vi "24HP_Convert serial string to Eng vals.vi"(0 "Serial buffer string (excluding FrameChar)":string) -> (2 "Pressures":sgl[][](graph), 3 "T_external (°C)":sgl format="%#_4f", 4 "T_board (°C)":sgl format="%#_4f", 6 "P_atmos (mbar)":sgl format="%#_4f", 8 "RH (%)":sgl format="%#_4f", 10 "a_xyz (g)":sgl[](array[numeric]), 13 "All vals":sgl[](array[numeric]), 14 "Status bytes":u8[](array[numeric]), 15 "w_xyz (deg/s)":sgl[](array[numeric]))   [LabVIEW 2020]
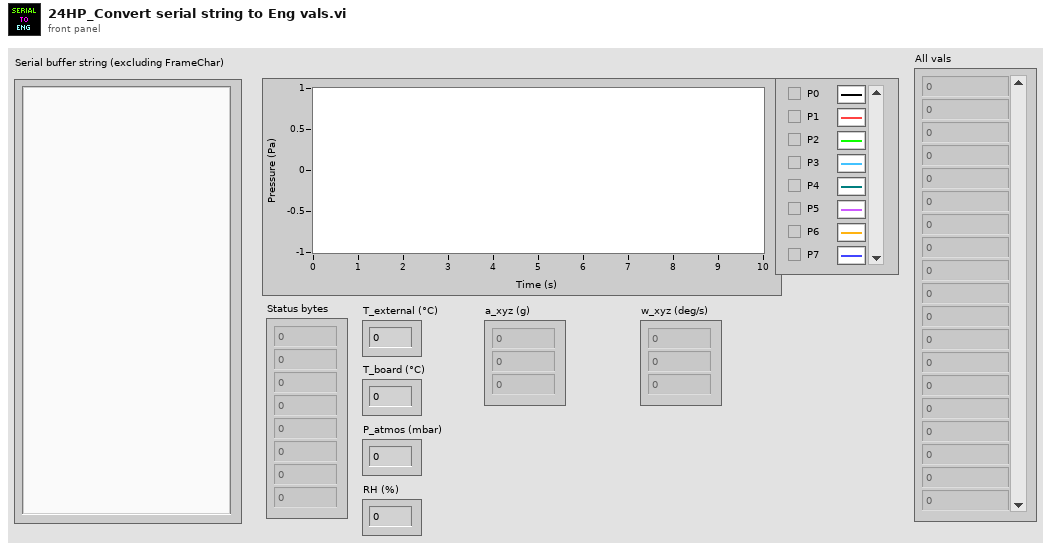
[diagram p1: front panel]
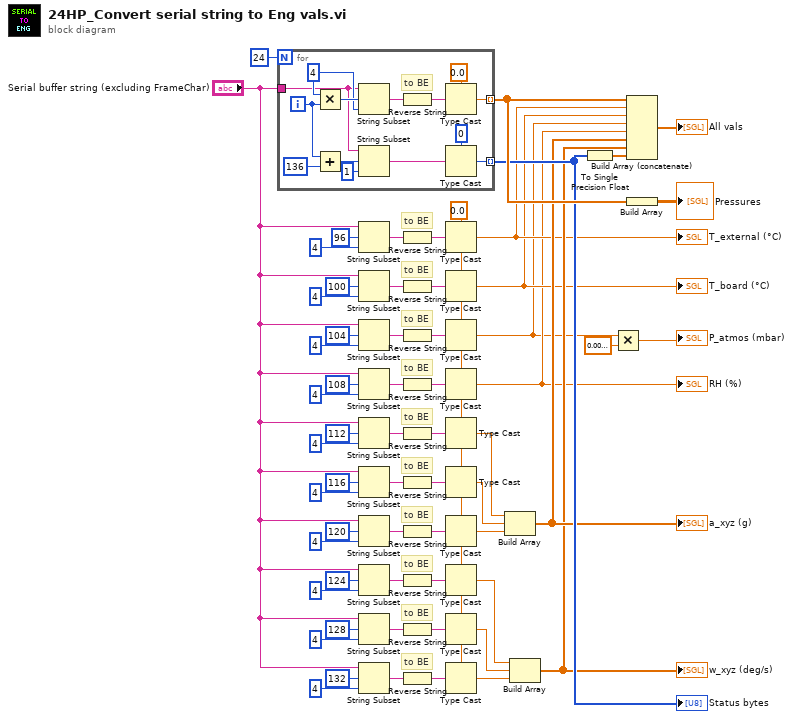
[diagram p0: block diagram]
diagram:
  w5 = sgl 0.0 ("byte count")
  # "to BE"
  # "to BE"
  # "to BE"
  # "to BE"
  # "to BE"
  # "to BE"
  # "to BE"
  # "to BE"
  # "to BE"
  # "to BE"
  n1 = for {
    N: 24 -> [_]
    tunnel: [w71] -> w60 mode=indexing
    tunnel: "Serial buffer string (excluding FrameChar)" -> [w67]
    tunnel: [w63] -> w59 mode=indexing
    i -> [w70]
    w75 = 4 ("x")
    # "to BE"
    n2 = Multiply(x=w75, y=w70) -> (x*y=w76:i32)
    n3 = Add(x=w70, y=136) -> (x+y=w68:i32)
    n4 = String Subset(string=w67, offset (0)=w76, length (rest)=w75) -> (substring=w74:string)
    n5 = String Subset(string=w67, offset (0)=w68, length (rest)=1 ("length (rest)")) -> (substring=w65:string)
    n6 = Reverse String(1:w74) -> (0:w73:string)
    n7 = Type Cast(type=sgl 0.0 ("byte count"), x=w73) -> (*(type *) &x=w71:sgl)
    n8 = Type Cast(type=u8 0 ("byte count"), x=w65) -> (*(type *) &x=w63:u8)
  }
  "Status bytes" <- w59
  n9 = String Subset(string="Serial buffer string (excluding FrameChar)", offset (0)=96, length (rest)=4 ("length (rest)")) -> (substring=w56:string)
  n10 = String Subset(string="Serial buffer string (excluding FrameChar)", offset (0)=100, length (rest)=4 ("length (rest)")) -> (substring=w51:string)
  n11 = String Subset(string="Serial buffer string (excluding FrameChar)", offset (0)=104, length (rest)=4 ("length (rest)")) -> (substring=w13:string)
  n12 = String Subset(string="Serial buffer string (excluding FrameChar)", offset (0)=108, length (rest)=4 ("length (rest)")) -> (substring=w8:string)
  n13 = String Subset(string="Serial buffer string (excluding FrameChar)", offset (0)=112, length (rest)=4 ("length (rest)")) -> (substring=w47:string)
  n14 = String Subset(string="Serial buffer string (excluding FrameChar)", offset (0)=116, length (rest)=4 ("length (rest)")) -> (substring=w42:string)
  n15 = String Subset(string="Serial buffer string (excluding FrameChar)", offset (0)=120, length (rest)=4 ("length (rest)")) -> (substring=w34:string)
  n16 = String Subset(string="Serial buffer string (excluding FrameChar)", offset (0)=124, length (rest)=4 ("length (rest)")) -> (substring=w39:string)
  n17 = String Subset(string="Serial buffer string (excluding FrameChar)", offset (0)=128, length (rest)=4 ("length (rest)")) -> (substring=w31:string)
  n18 = String Subset(string="Serial buffer string (excluding FrameChar)", offset (0)=132, length (rest)=4 ("length (rest)")) -> (substring=w26:string)
  n19 = Reverse String(1:w56) -> (0:w57:string)
  n20 = Reverse String(1:w51) -> (0:w50:string)
  n21 = Reverse String(1:w13) -> (0:w14:string)
  n22 = Reverse String(1:w8) -> (0:w7:string)
  n23 = Reverse String(1:w47) -> (0:w48:string)
  n24 = Reverse String(1:w42) -> (0:w41:string)
  n25 = Reverse String(1:w34) -> (0:w33:string)
  n26 = Reverse String(1:w39) -> (0:w40:string)
  n27 = Reverse String(1:w31) -> (0:w32:string)
  n28 = Reverse String(1:w26) -> (0:w25:string)
  n29 = Type Cast(type=w5, x=w57) -> (*(type *) &x=w16:sgl)
  "T_external (°C)" <- w16
  n30 = Type Cast(type=w5, x=w50) -> (*(type *) &x=w15:sgl)
  "T_board (°C)" <- w15
  n31 = Type Cast(type=w5, x=w14) -> (*(type *) &x=w2:sgl)
  n32 = Type Cast(type=w5, x=w7) -> (*(type *) &x=w4:sgl)
  "RH (%)" <- w4
  n33 = Type Cast(type=w5, x=w48) -> (*(type *) &x=w24:sgl)
  n34 = Type Cast(type=w5, x=w41) -> (*(type *) &x=w23:sgl)
  n35 = Type Cast(type=w5, x=w33) -> (*(type *) &x=w22:sgl)
  n36 = Type Cast(type=w5, x=w40) -> (*(type *) &x=w21:sgl)
  n37 = Type Cast(type=w5, x=w32) -> (*(type *) &x=w20:sgl)
  n38 = Type Cast(type=w5, x=w25) -> (*(type *) &x=w19:sgl)
  n39 = Build Array(w24, w23, w22) -> (w18:sgl[])
  "a_xyz (g)" <- w18
  n40 = Build Array(w21, w20, w19) -> (w17:sgl[])
  "w_xyz (deg/s)" <- w17
  n41 = To Single Precision Float(number=w59) -> (single precision float=w49:sgl[])
  n42 = Multiply(x=w2, y=sgl 0.01) -> (x*y=→"P_atmos (mbar)":sgl)
  n43 = Build Array (concatenate)(w60, w16, w15, w2, w4, w18, w17, w49) -> (→"All vals":sgl[])
  n44 = Build Array(w60) -> (→"Pressures":sgl[][])
